vi "Read Report Path.vi"(8 "error in (no error)":errorcluster, 11 "Report Information in":refnum<class "Report Information.lvclass">) -> (0 "error out":errorcluster, 2 "Report Path":path, 3 "Report Information out":refnum<class "Report Information.lvclass">)   [LabVIEW 2015, in "Report Information.lvclass"]
uses:
  Report Information.lvclass
  Report Information.lvclass/Report Information.ctl
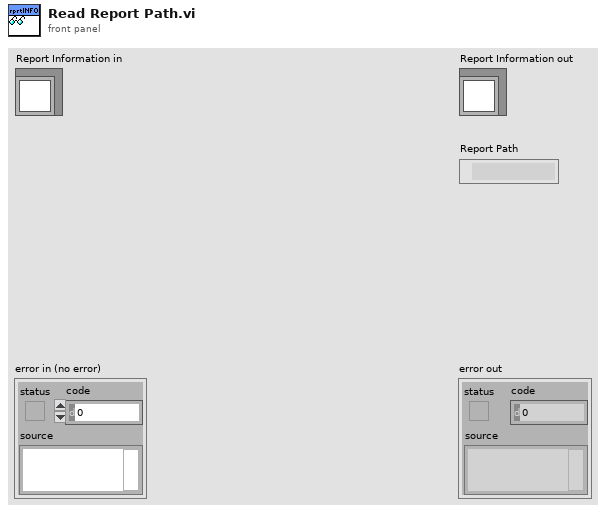
[diagram p1: front panel]
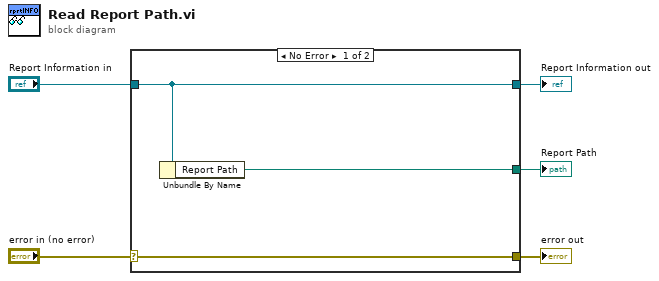
[diagram p0: block diagram]
diagram:
  n1 = case shown="No Error" "error in (no error)" {
    selector: "error in (no error)" -> [w8 w9]
    tunnel: [w8 w9] -> w4
    tunnel: [w7 w10] -> w2
    tunnel: "Report Information in" -> [w7 w10]
    tunnel: [w6 _] -> w1
    frame No Error {
      n2 = Unbundle By Name(w7) -> ("Report Path"=w6:path)
    }
    frame Error {
    }
  }
  "error out" <- w4
  "Report Information out" <- w2
  "Report Path" <- w1
